vi "onTestDiscovery.vi"(8 "error in (no error)":errorcluster, 11 "Test Runner.Collection in":refnum<class "Test Runner.Collection.lvclass">) -> (0 "error out":errorcluster, 2 "Tests VIs":path[](array[path]), 3 "Test Runner.Collection out":refnum<class "Test Runner.Collection.lvclass">)   [LabVIEW 2013, in "Caraya.lvlib" / "Test Runner.Collection.lvclass"]
uses:
  Test Runner.Collection.lvclass
  Test Runner.Collection.lvclass/Test Runner.Collection.ctl
  Test Runner/Test Runner.lvclass
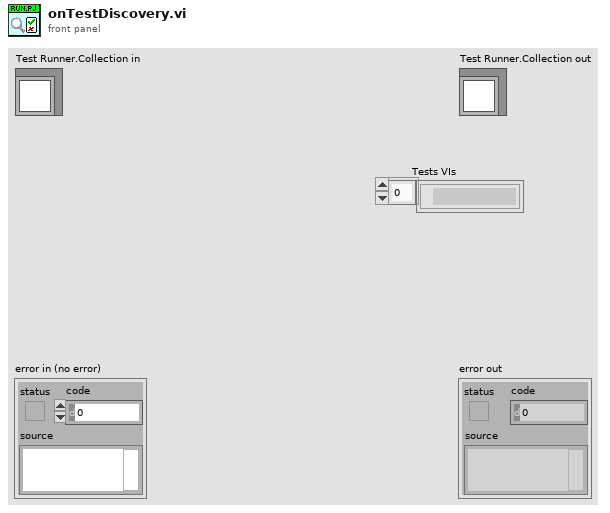
[diagram p1: front panel]
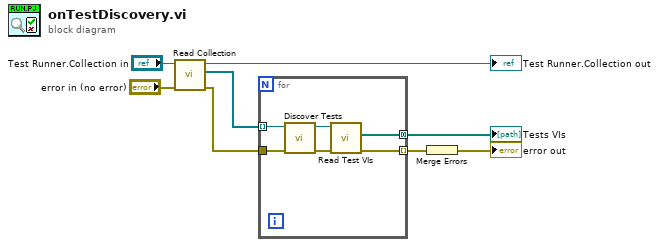
[diagram p0: block diagram]
diagram:
  n1 = call "Read Collection.vi"("error in (no error)"="error in (no error)", "Test Runner.Collection in"="Test Runner.Collection in") -> ("error out"=w4:errorcluster, "Test Runners"=w2:refnum<class "Test Runner.lvclass">[], "Test Runner.Collection out"=→"Test Runner.Collection out":refnum<class "Test Runner.Collection.lvclass">)  [unwired: 7 in]
  n2 = for {
    tunnel: [w10] -> w7 mode=concatenating
    tunnel: w2 -> [w9] mode=indexing
    tunnel: w4 -> [w14]
    tunnel: [w11] -> w8 mode=indexing
    n3 = call "Discover Tests.vi"("error in (no error)"=w14, "Test Runner in"=w9) -> ("error out"=w12:errorcluster, "Test Runner out"=w13:refnum<class "Test Runner.lvclass">)  [unwired: 8 in]
    n4 = call-dynamic "Read Test VIs.vi"("error in (no error)"=w12, "Test Runner in"=w13) -> ("error out"=w11:errorcluster, "Test VIs"=w10:path[])  [unwired: 7 in, 1 out]
  }
  "Tests VIs" <- w7
  n5 = Merge Errors(w8) -> (→"error out":errorcluster)
